vi "OCB_PositionSelector.vi"(2 "OCB Enable":bool, 3 "OperatorControlBox Buttons":T2) -> (0 "NewPosition":bool, 1 "OCB Latest Position":T1)   [LabVIEW 2018]
uses:
  TypeDefs/OperatorControlBoxButtons_Type.ctl
  TypeDefs/OperatorControlBoxButtonPosition_Type.ctl
  ArgosLib/Signal Processing/TypeDefs/EdgeDetector_Type.ctl
  ArgosLib/ArgosLib.lvlib
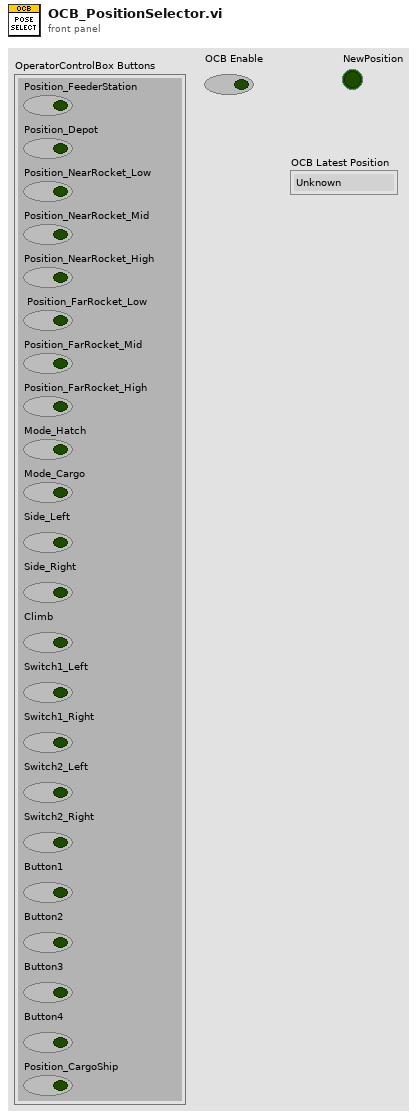
[diagram p1: front panel]
types:
  T1 = typedef "OperatorControlBoxButtonPosition_Type.ctl" = enum16{"Unknown", "FeederStation", "Depot", "NearRocketLow", "NearRocketMid", "NearRocketHigh", "FarRocketLow", "FarRocketMid", "FarRocketHigh", "CargoShip"}
  T2 = typedef "OperatorControlBoxButtons_Type.ctl" = cluster{"Position_FeederStation":bool, "Position_Depot":bool, "Position_NearRocket_Low":bool, "Position_NearRocket_Mid":bool, "Position_NearRocket_High":bool, " Position_FarRocket_Low":bool, "Position_FarRocket_Mid":bool, "Position_FarRocket_High":bool, "Mode_Hatch":bool, "Mode_Cargo":bool, "Side_Left":bool, "Side_Right":bool, "Climb":bool, "Switch1_Left":bool, "Switch1_Right":bool, "Switch2_Left":bool, "Switch2_Right":bool, "Button1":bool, "Button2":bool, "Button3":bool, "Button4":bool, "Position_CargoShip":bool}
  T3 = typedef "ArgosLib.lvlib/EdgeDetector_Type.ctl" = enum16{"RisingEdge", "FallingEdge", "Both"}
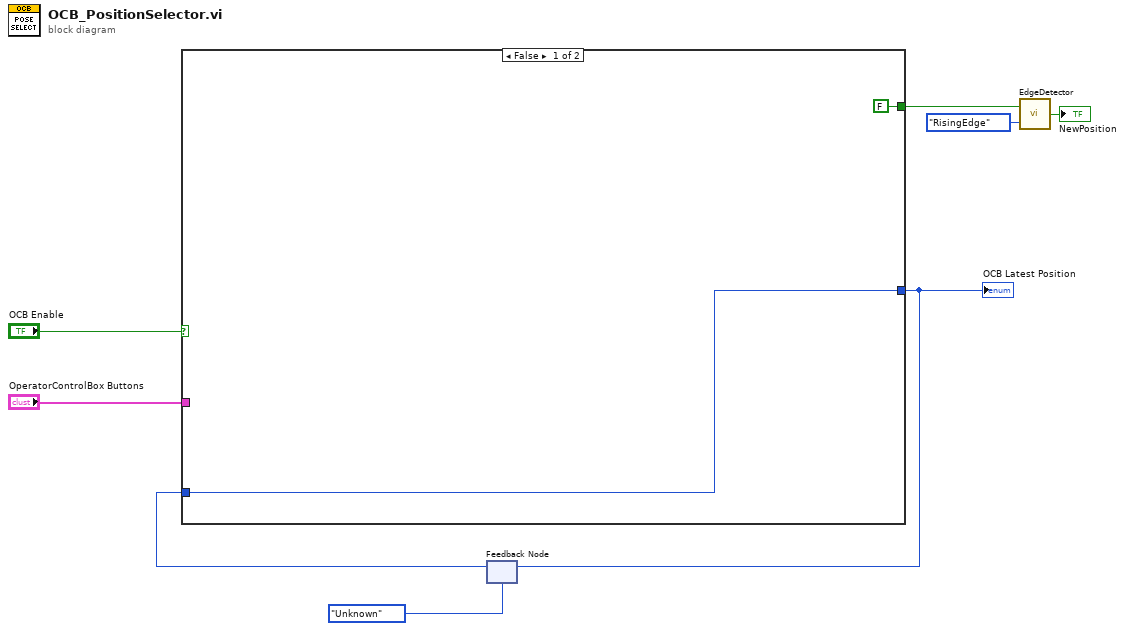
[diagram p0: block diagram]
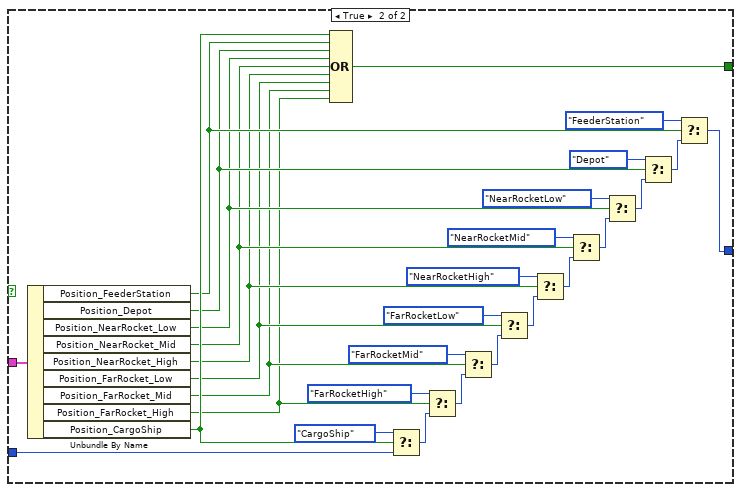
[diagram p2: hidden frame]
diagram:
  n1 = feedback #1(OperatorControlBoxButtonPosition_Type."Unknown" ("OCB Latest Position")) -> (w6:T1)
  n2 = case shown="False" "OCB Enable" {
    tunnel: "OperatorControlBox Buttons" -> [_ w40]
    tunnel: w6 -> [w10 w39]
    tunnel: [w10 w30] -> w5
    tunnel: [FALSE w11] -> w3
    frame False {
    }
    frame True {
      n3 = Unbundle By Name(w40) -> ("Position_FeederStation"=w19:bool, "Position_Depot"=w18:bool, "Position_NearRocket_Low"=w17:bool, "Position_NearRocket_Mid"=w16:bool, "Position_NearRocket_High"=w15:bool, "Position_FarRocket_Low"=w14:bool, "Position_FarRocket_Mid"=w13:bool, "Position_FarRocket_High"=w12:bool, "Position_CargoShip"=w20:bool)
      n4 = Compound Arithmetic op=OR(w20, w19, w18, w17, w16, w15, w14, w13, w12) -> (w11:bool)
      n5 = Select(t=OperatorControlBoxButtonPosition_Type."CargoShip", s=w20, f=w39) -> (s? t:f=w38:T1)
      n6 = Select(t=OperatorControlBoxButtonPosition_Type."FarRocketHigh", s=w12, f=w38) -> (s? t:f=w37:T1)
      n7 = Select(t=OperatorControlBoxButtonPosition_Type."FarRocketMid", s=w13, f=w37) -> (s? t:f=w36:T1)
      n8 = Select(t=OperatorControlBoxButtonPosition_Type."FarRocketLow", s=w14, f=w36) -> (s? t:f=w35:T1)
      n9 = Select(t=OperatorControlBoxButtonPosition_Type."NearRocketHigh", s=w15, f=w35) -> (s? t:f=w34:T1)
      n10 = Select(t=OperatorControlBoxButtonPosition_Type."NearRocketMid", s=w16, f=w34) -> (s? t:f=w33:T1)
      n11 = Select(t=OperatorControlBoxButtonPosition_Type."NearRocketLow", s=w17, f=w33) -> (s? t:f=w32:T1)
      n12 = Select(t=OperatorControlBoxButtonPosition_Type."Depot", s=w18, f=w32) -> (s? t:f=w31:T1)
      n13 = Select(t=OperatorControlBoxButtonPosition_Type."FeederStation", s=w19, f=w31) -> (s? t:f=w30:T1)
    }
  }
  "OCB Latest Position" <- w5
  n14 = feedback-in #1(w5) -> ()
  n15 = call "EdgeDetector.vi"("DetectorType"=EdgeDetector_Type."RisingEdge", "Input"=w3) -> ("Edge"=→"NewPosition":bool)
